vi "配置文件路径.vi"(11 "TimingControl 输入":refnum<class "TimingControl.lvclass">) -> (3 "TimingControl 输出":refnum<class "TimingControl.lvclass">)   [LabVIEW 2016, in "TimingControl.lvclass"]
uses:
  TimingControl.lvclass
  TimingControl.lvclass/TimingControl.ctl
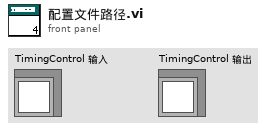
[diagram p1: front panel]
types:
  T1 = typedef "TimingControl.lvclass/State Data.ctl" = cluster{"仪器时间":timestamp, "仪器运行状态":bool, "配置文件路径":path, "测量参数":u16, "测试状态":cluster{"启动时间":timestamp, "结束时间":timestamp, "启动次数":dbl}, "配置信息":cluster{"每周启动":T2, "每月启动":T3, "周期模式":T4, "测量参数":T5, "定点周期":T6, "间隔启动":T8}}
  T2 = typedef "TimingControl.lvclass/每周启动.ctl" = enum16{"关闭", "周日", "周一", "周二", "周三", "周四", "周五", "周六"}
  T3 = typedef "TimingControl.lvclass/每月启动.ctl" = enum16{"关闭", "1号", "2号", "3号", "4号", "5号", "6号", "7号", "8号", "9号", "10号", "11号", "12号", "13号", "14号", "15号", "16号", "17号", "18号", "19号", "20号", "21号", "22号", "23号", "24号", "25号", "26号", "27号", "28号", "29号", "30号", "31号"}
  T4 = typedef "TimingControl.lvclass/周期模式设置.ctl" = enum16{"不启用", "定点模式", "间隔模式"}
  T5 = typedef "TimingControl.lvclass/测量参数.ctl" = u16
  T6 = typedef "TimingControl.lvclass/定点周期设置.ctl" = cluster{"启动命令":T7, "启动命令 2":T7, "启动命令 3":T7, "启动命令 4":T7, "启动命令 5":T7, "启动命令 6":T7, "启动命令 7":T7, "启动命令 8":T7, "启动命令 9":T7, "启动命令 10":T7, "启动命令 11":T7, "启动命令 12":T7, "启动命令 13":T7, "启动命令 14":T7, "启动命令 15":T7, "启动命令 16":T7, "启动命令 17":T7, "启动命令 18":T7, "启动命令 19":T7, "启动命令 20":T7, "启动命令 21":T7, "启动命令 22":T7, "启动命令 23":T7, "启动命令 24":T7}
  T7 = typedef "TimingControl.lvclass/启动命令选择.ctl" = enum16{"", "水样测试", "标样核查", "零点核查", "跨度核查", "空白测试", "平行样测试", "加标回收", "空白校准", "标样校准", "初始化(清洗)"}
  T8 = typedef "TimingControl.lvclass/间隔启动设置.ctl" = cluster{"启动命令":T7, "启动间隔":dbl, "启动次数":i32}
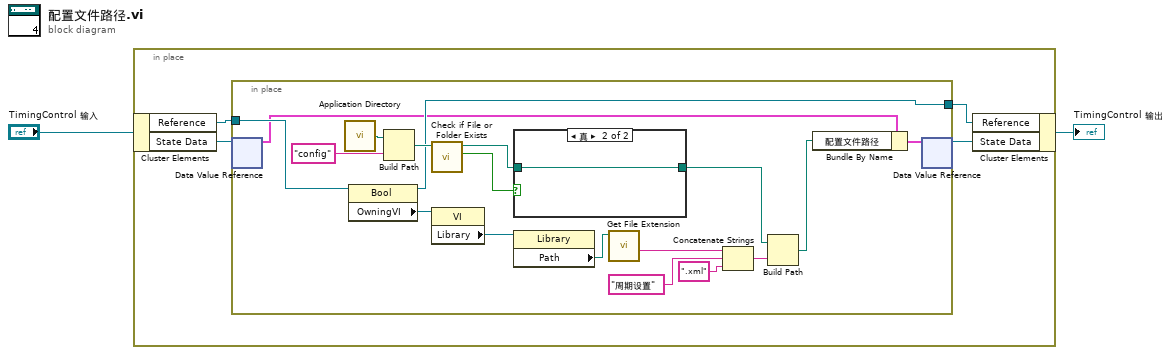
[diagram p0: block diagram]
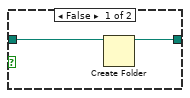
[diagram p2: hidden frame]
diagram:
  n1 = in-place {
    n2 = in-place-cluster #1("TimingControl 输入") -> ("Reference"=w6:refnum<vi>, "State Data"=w4:refnum<data-value>)
    n3 = in-place {
      in-place-border: w6 -> [w13]
      in-place-border: [w12] -> w5
      n4 = in-place-dvr #2(w4) -> (w11:T1)  [unwired: 1 out]
      n5 = call <vilib>:"Application Directory.vi"() -> ("Application Directory"=w21:path)
      n6 = property class="Bool"(reference=w13) -> (reference out=w12:refnum<vi>, "OwningVI"=w23:refnum<vi>)  [unwired: 1 in, 1 out]
      n7 = Build Path(base path=w21, name or relative path="config" ("名称或相对路径")) -> (appended path=w19:path)
      n8 = call <vilib>:"Check if File or Folder Exists.vi"("path"=w19) -> ("file or folder exists?"=w16:bool, "dup path"=w15:path)  [unwired: 8 in, 1 out]
      n9 = property class="VI"(reference=w23) -> ("Library"=w24:refnum<vi>)  [unwired: 1 in, 2 out]
      n10 = case shown="真" w16 {
        tunnel: w15 -> [w26 w27]
        tunnel: [w25 w27] -> w14
        frame False {
          n11 = Create Folder(path (use dialog)=w26) -> (created path=w25:path)  [unwired: 2 in, 2 out]
        }
        frame True {
        }
      }
      n12 = property class="Library"(reference=w24) -> ("Path"=w22:path)  [unwired: 1 in, 2 out]
      n13 = call <vilib>:"Get File Extension.vi"("file"=w22) -> ("filename without extension"=w8:string)  [unwired: 6 in, 4 out]
      n14 = Concatenate Strings(w8, "周期设置" ("字符串"), ".xml" ("字符串")) -> (w17:string)
      n15 = Build Path(base path=w14, name or relative path=w17) -> (appended path=w9:path)
      n16 = Bundle By Name(cluster=w11, "配置文件路径"=w9) -> (w10:T1)
      n17 = in-place-dvr #2(w10) -> (w3:refnum<data-value>)  [unwired: 1 out]
    }
    n18 = in-place-cluster #1("Reference"=w5, "State Data"=w3) -> (→"TimingControl 输出":refnum<class "TimingControl.lvclass">)
  }
